vi "test Uninitialized Instance.vi"(8 "error in":errorcluster) -> (0 "error out":errorcluster)   [LabVIEW 2024, in "serenial.io-ase.test.lvlib"]
uses:
  serenial.io-ase.test.lvlib
  serenial.io-ase/ase/ase.lvclass
  <vilib>/addons/_JKI Toolkits/Caraya/classes/Test/Test.lvclass
  <vilib>/addons/_JKI Toolkits/Caraya/classes/Assert/Assert.lvclass
  <vilib>/addons/_JKI Toolkits/Caraya/classes/Assert/Assert Equal Value and Type_Variant.vi
  serenial.io-ase/ase/Call State.ctl
  serenial.io-ase/ase/Standard Input State.ctl
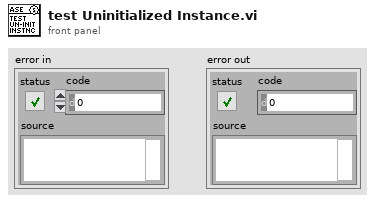
[diagram p1: front panel]
types:
  T1 = typedef "serenial.io-ase.lvlib/ase.lvclass/Standard Input State.ctl" = enum16{"Open/Closing", "Closed"}
  T2 = typedef "serenial.io-ase.lvlib/ase.lvclass/Call State.ctl" = enum16{"Running/Terminating", "Already Exited"}
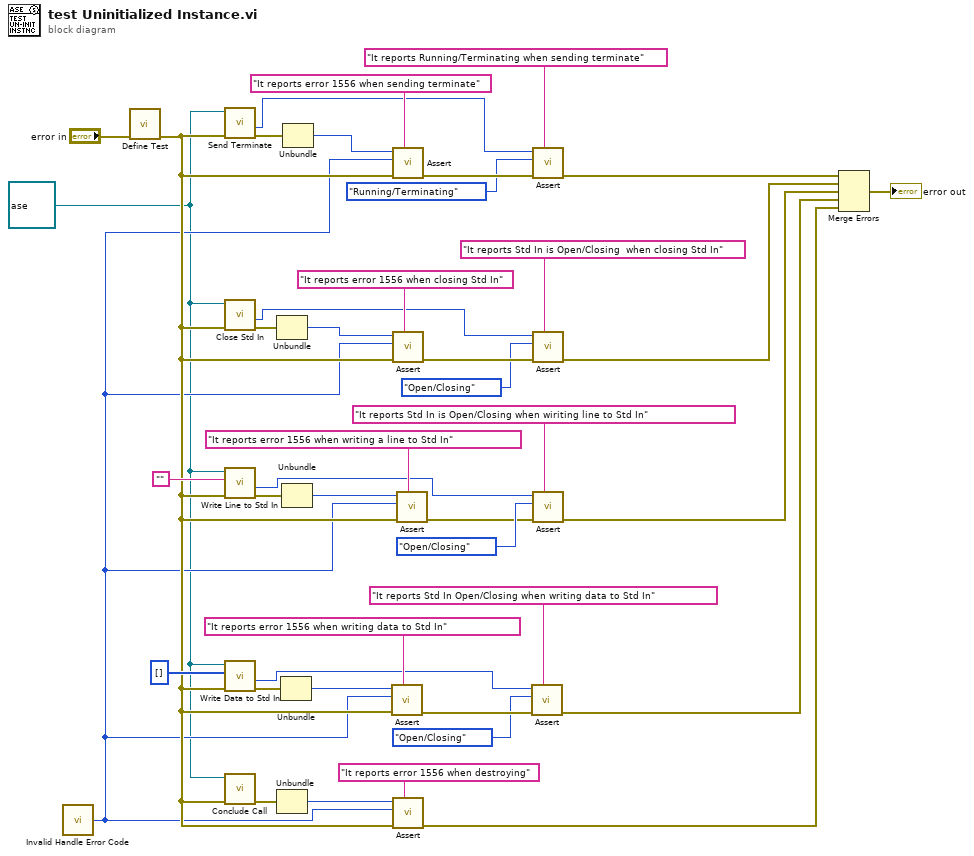
[diagram p0: block diagram]
diagram:
  w1 = refnum<class "ase.lvclass"> refnum ("serenial.io-ase.lvlib:serenial.io-ase.lvclass")
  n1 = call "Invalid Handle Error Code.vi"() -> ("Invalid Handle Error"=w2:i32)
  n2 = call <vilib>:"Define Test.vi"("error in (no error)"="error in") -> ("error out"=w13:errorcluster)  [unwired: 9 in, 1 out]
  n3 = call "Send Terminate.vi"("error in"=w13, "ASE Handle"=w1) -> ("error out"=w31:errorcluster, "State"=w19:T2)  [unwired: 7 in, 1 out]
  n4 = call "Close Std In.vi"("error in"=w13, "ASE Handle"=w1) -> ("error out"=w33:errorcluster, "State"=w18:T1)  [unwired: 7 in, 1 out]
  n5 = call "Write Line to Std In .vi"("error in"=w13, "Input"="", "ASE Handle"=w1) -> ("error out"=w43:errorcluster, "State"=w25:T1)  [unwired: 6 in, 1 out]
  n6 = call "Write Data to Std In.vi"("error in"=w13, "Data"=u8[] [], "ASE Handle"=w1) -> ("error out"=w34:errorcluster, "State"=w9:T1)  [unwired: 6 in, 1 out]
  n7 = call "Conclude Call.vi"("error in"=w13, "ASE Handle"=w1) -> ("error out"=w24:errorcluster)  [unwired: 7 in, 2 out]
  n8 = Unbundle(w33) -> ("code"=w32:i32)  [unwired: 2 out]
  n9 = Unbundle(w24) -> ("code"=w23:i32)  [unwired: 2 out]
  n10 = Unbundle(w34) -> ("code"=w14:i32)  [unwired: 2 out]
  n11 = Unbundle(w43) -> ("code"=w16:i32)  [unwired: 2 out]
  n12 = Unbundle(w31) -> ("code"=w30:i32)  [unwired: 2 out]
  n13 = call-poly <vilib>:"Assert.vi"("Label"="It reports error 1556 when writing data to Std In", "error in (no error)"=w13, "Y"=w2, "X"=w14) -> ("error out"=w11:errorcluster)  [unwired: 6 in, 1 out]
  n14 = call-poly <vilib>:"Assert.vi"("Label"="It reports error 1556 when sending terminate", "error in (no error)"=w13, "Y"=w2, "X"=w30) -> ("error out"=w36:errorcluster)  [unwired: 6 in, 1 out]
  n15 = call-poly <vilib>:"Assert.vi"("Label"="It reports error 1556 when closing Std In", "error in (no error)"=w13, "Y"=w2, "X"=w32) -> ("error out"=w29:errorcluster)  [unwired: 6 in, 1 out]
  n16 = call-poly <vilib>:"Assert.vi"("Label"="It reports error 1556 when destroying", "error in (no error)"=w13, "Y"=w2, "X"=w23) -> ("error out"=w4:errorcluster)  [unwired: 6 in, 1 out]
  n17 = call-poly <vilib>:"Assert.vi"("Label"="It reports error 1556 when writing a line to Std In", "error in (no error)"=w13, "Y"=w2, "X"=w16) -> ("error out"=w12:errorcluster)  [unwired: 6 in, 1 out]
  n18 = call-poly <vilib>:"Assert.vi"("Label"="It reports Std In Open/Closing when writing data to Std In", "error in (no error)"=w11, "Y"=Standard_Input_State."Open/Closing" ("State"), "X"=w9) -> ("error out"=w5:errorcluster)  [unwired: 6 in, 1 out]
  n19 = call-poly <vilib>:"Assert.vi"("Label"="It reports Running/Terminating when sending terminate", "error in (no error)"=w36, "Y"=Call_State."Running/Terminating" ("State"), "X"=w19) -> ("error out"=w8:errorcluster)  [unwired: 6 in, 1 out]
  n20 = call-poly <vilib>:"Assert.vi"("Label"="It reports Std In is Open/Closing  when closing Std In", "error in (no error)"=w29, "Y"=Standard_Input_State."Open/Closing" ("State"), "X"=w18) -> ("error out"=w7:errorcluster)  [unwired: 6 in, 1 out]
  n21 = call-poly <vilib>:"Assert.vi"("Label"="It reports Std In is Open/Closing when wiriting line to Std In", "error in (no error)"=w12, "Y"=Standard_Input_State."Open/Closing" ("State"), "X"=w25) -> ("error out"=w6:errorcluster)  [unwired: 6 in, 1 out]
  n22 = Merge Errors(w8, w7, w6, w5, w4) -> (→"error out":errorcluster)
